vi "Set Parent Values from Template.vi"(0 "template configuration":refnum<class "SV Signal.lvclass">, 2 "signal configuration in":refnum<class "SV Function.lvclass">, 7 "error in (no error)":errorcluster) -> (4 "signal configuration out":refnum<class "SV Function.lvclass">, 6 "template used?":bool, 8 "error out":errorcluster)   [LabVIEW 2017, in "SV Function.lvclass"]
uses:
  <vilib>/addons/_NISVFA/_Generation/Signal Generation/SV Function/SV Function.lvclass
  <vilib>/addons/_NISVFA/_Generation/Signal Generation/SV Signal/SV Signal.lvclass
  <vilib>/addons/_NISVFA/_Generation/Signal Generation/SV Function/SV Function.lvclass/SV Function.ctl
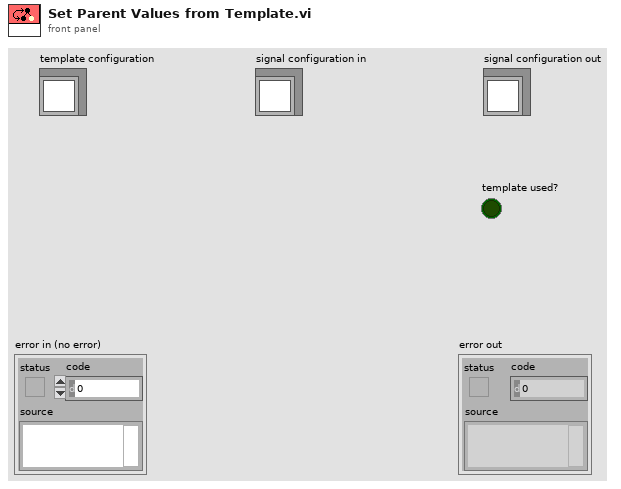
[diagram p1: front panel]
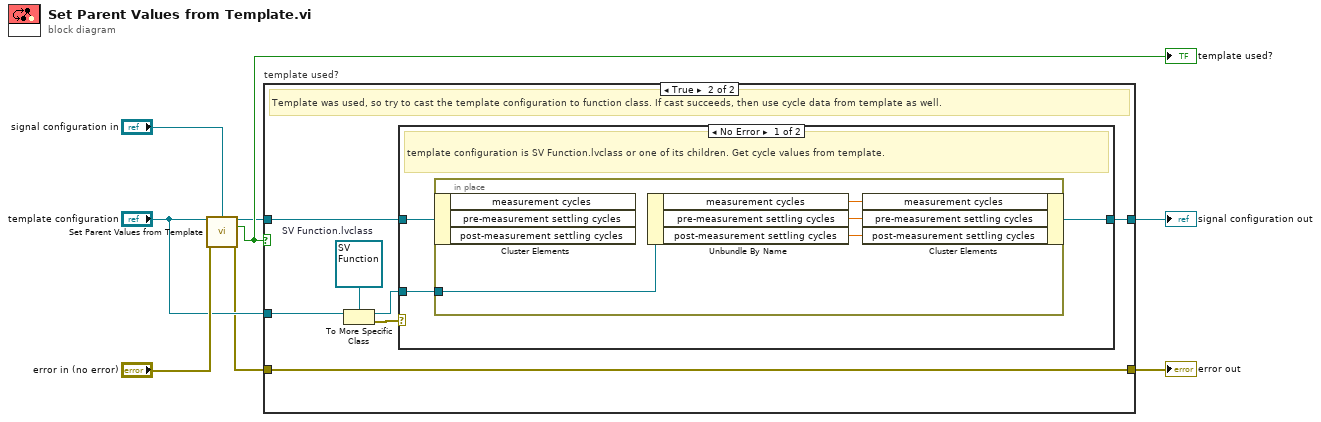
[diagram p0: block diagram]
diagram:
  n1 = call-parent "Set Parent Values from Template.vi"("template configuration"="template configuration", "signal configuration in"="signal configuration in", "error in (no error)"="error in (no error)") -> ("signal configuration out"=w2:refnum<class "SV Function.lvclass">, "template used?"=w3:bool, "error out"=w5:errorcluster)  [unwired: 10 in]
  "template used?" <- w3
  n2 = case "template used?" shown="True" w3 {
    tunnel: "template configuration" -> [_ w17]
    tunnel: w5 -> [w9 w15]
    tunnel: [w9 w15] -> w4
    tunnel: w2 -> [w10 w11]
    tunnel: [w10 w12] -> w1
    frame False {
      # "Template was not used. There is no need to write any additional template information to the main configuration"
    }
    frame True {
      w16 = refnum<class "SV Function.lvclass"> refnum  # SV Function.lvclass
      # "Template was used, so try to cast the template configuration to function class. If cast succeeds, then use cycle data from template as well."
      n3 = To More Specific Class(target class=w16, reference=w17) -> (specific class reference=w13:refnum<class "SV Function.lvclass">, error out=w14:errorcluster)  [unwired: 1 in]
      n4 = case shown="No Error" w14 {
        tunnel: w13 -> [w20 _]
        tunnel: [w18 w25] -> w12
        tunnel: w11 -> [w19 w25]
        frame No Error {
          # "template configuration is SV Function.lvclass or one of its children. Get cycle values from template."
          n5 = in-place {
            in-place-border: w20 -> [w24]
            n6 = in-place-cluster #1(w19) -> ()  [unwired: 3 out]
            n7 = Unbundle By Name(w24) -> ("measurement cycles"=w23:dbl, "pre-measurement settling cycles"=w22:dbl, "post-measurement settling cycles"=w21:dbl)
            n8 = in-place-cluster #1("measurement cycles"=w23, "pre-measurement settling cycles"=w22, "post-measurement settling cycles"=w21) -> (w18:refnum<class "SV Function.lvclass">)
          }
        }
        frame Error {
          # "To More Specific Class errored, so template configuration is not SV Function.lvclass or one of its children. No need to set additional values."
        }
      }
    }
  }
  "error out" <- w4
  "signal configuration out" <- w1
